vi "GetTetColors.vi"(8 "error in (no error)":errorcluster, 11 "DisplayTetrodes in":refnum<class "DisplayTetrodes.lvclass">=refnum) -> (0 "error out":errorcluster, 1 "Photodiode":u32(colorbox)=16514929, 2 "Tet Colors":u32[](array[numeric])=[16718354, 3669778, 2792191, 16711925, 16772882, 2780, 1245167, 16741650, 2504, 13874861, 10813184, 16769536, 42751, 14090495, 35200, 13565696, 16735744, 6755071, 51283, 14090168, 16318719, 24575, 11837952, 7012552, 10650492, 10420233, 19932, 1228799], 3 "DisplayTetrodes out":refnum<class "DisplayTetrodes.lvclass">)   [LabVIEW 2010, in "DisplayTetrodes.lvclass"]
uses:
  DisplayTetrodes.lvclass
panel:
  in  "Photodiode":u32(colorbox)=16514929
  in  "Tet 28":u32(colorbox)=16514929
  in  "Tet 27":u32(colorbox)=16775072
  in  "Tet 26":u32(colorbox)=10420233
  in  "Tet 25":u32(colorbox)=16448250
  in  "Tet 24":u32(colorbox)=7012552
  in  "Tet 23":u32(colorbox)=11837952
  in  "Tet 22":u32(colorbox)=24575
  in  "Tet 21":u32(colorbox)=16318719
  in  "Tet 20":u32(colorbox)=16448250
  in  "Tet 19":u32(colorbox)=51283
  in  "Tet 18":u32(colorbox)=6755071
  in  "Tet 17":u32(colorbox)=16735744
  in  "Tet 16":u32(colorbox)=13565696
  in  "Tet 15":u32(colorbox)=16448250
  in  "Tet 14":u32(colorbox)=14090495
  in  "Tet 13":u32(colorbox)=42751
  in  "Tet 12":u32(colorbox)=16769536
  in  "Tet 11":u32(colorbox)=10813184
  in  "Tet 10":u32(colorbox)=16448250
  in  "Tet 9":u32(colorbox)=2504
  in  "Tet 8":u32(colorbox)=16741650
  in  "Tet 7":u32(colorbox)=1245167
  in  "Tet 6":u32(colorbox)=2780
  in  "Tet 5":u32(colorbox)=16448250
  in  "Tet 4":u32(colorbox)=16711925
  in  "Tet 3":u32(colorbox)=2792191
  in  "Tet 2":u32(colorbox)=3669778
  in  "Tet 1":u32(colorbox)=16448250
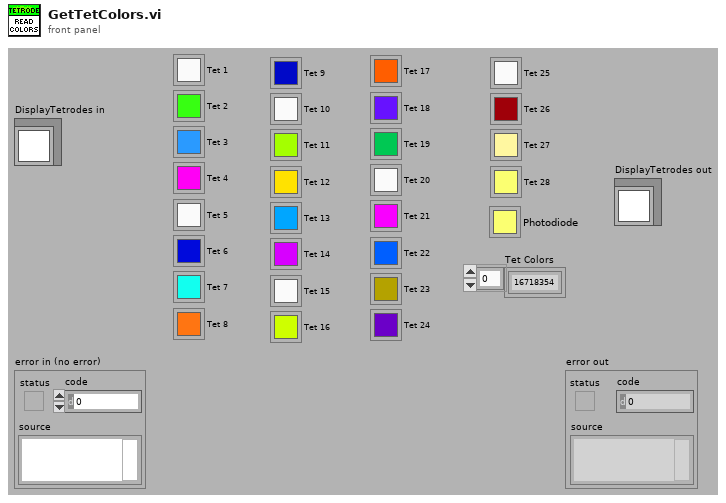
[diagram p1: front panel]
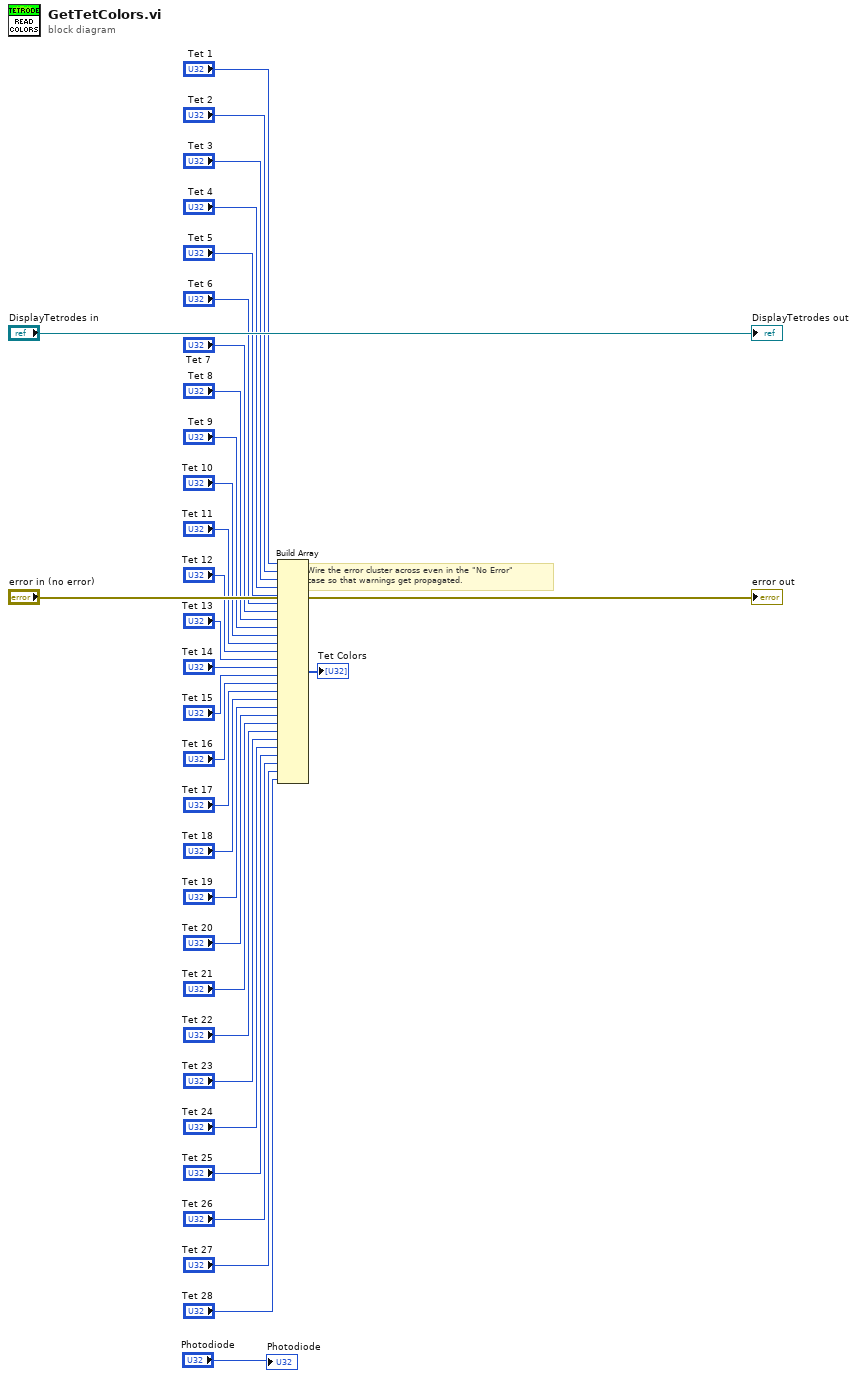
[diagram p0: block diagram]
diagram:
  # "Wire the error cluster across even in the \"No Error\"\ncase so that warnings get propagated."
  n1 = Build Array("Tet 1", "Tet 2", "Tet 3", "Tet 4", "Tet 5", "Tet 6", "Tet 7", "Tet 8", "Tet 9", "Tet 10", "Tet 11", "Tet 12", "Tet 13", "Tet 14", "Tet 15", "Tet 16", "Tet 17", "Tet 18", "Tet 19", "Tet 20", "Tet 21", "Tet 22", "Tet 23", "Tet 24", "Tet 25", "Tet 26", "Tet 27", "Tet 28") -> (→"Tet Colors":u32[])
  "error out" <- "error in (no error)"
  "DisplayTetrodes out" <- "DisplayTetrodes in"
  "Photodiode" <- "Photodiode"
